vi "seguidor_parede_odometria.vi"(3 "Text":string, 4 "Line":i16(ring) items=["1", "2", "3", "4", "5", "6", "7", "8", "9", "10", "11", "12"], 5 "NXT/EV3 3":T1) -> (0 "Numeric 2":i32, 2 "NXT/EV3 2":T1)   [LabVIEW 2016]
uses:
  <vilib>/NXT/Subs/LVHSConnector.ctl
  <vilib>/NXT/LegoClasses/BrickReference/BrickReference.lvclass
  <vilib>/NXT/Block Support/NXT_OutputPort.ctl
  <vilib>/NXT/Block Support/NXT_InputPort.ctl
  <vilib>/NXT/Dual Mode Library/Motors/ResetMotor.vi
  <vilib>/NXT/NXTIO Xnodes/NXTIONodeSubVIs/NXTMoveMotors.vi
  <vilib>/NXT/Dual Mode Library/Sensors/EV3_Ultrasonic_CM.vi
  <vilib>/NXT/Dual Mode Library/Sensors/Touch_Pressed.vi
  <vilib>/NXT/Dual Mode Library/Motors/Rotation.vi
  <vilib>/NXT/Dual Mode Library/Display/drawText.vi
  <vilib>/NXT/Dual Mode Library/Display/drawNumber_float.vi
  <vilib>/NXT/NXTIO Xnodes/AddressXNode/NXTIOAddress.xnode
  <vilib>/NXT/NXTIO Xnodes/NXTIOXNode/NXTIO.xnode
panel:
  in  "KE 2":dbl=-0.0356
  in  "Kp":sgl
  in  "Dmin":sgl
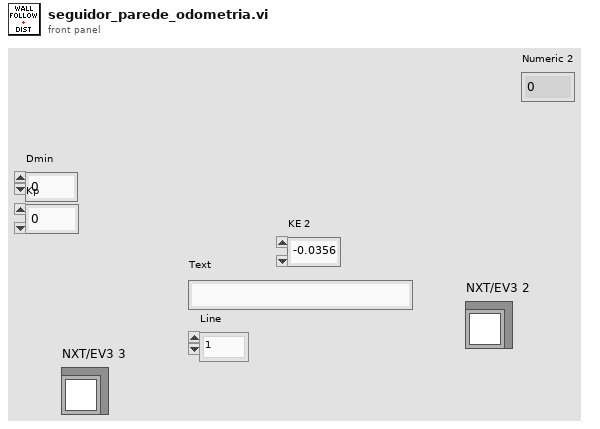
[diagram p1: front panel]
types:
  T1 = typedef "LVHSConnector.ctl" = refnum<class "BrickReference.lvclass">
  T2 = typedef "NXT_OutputPort.ctl" = u8
  T3 = typedef "NXT_InputPort.ctl" = u32
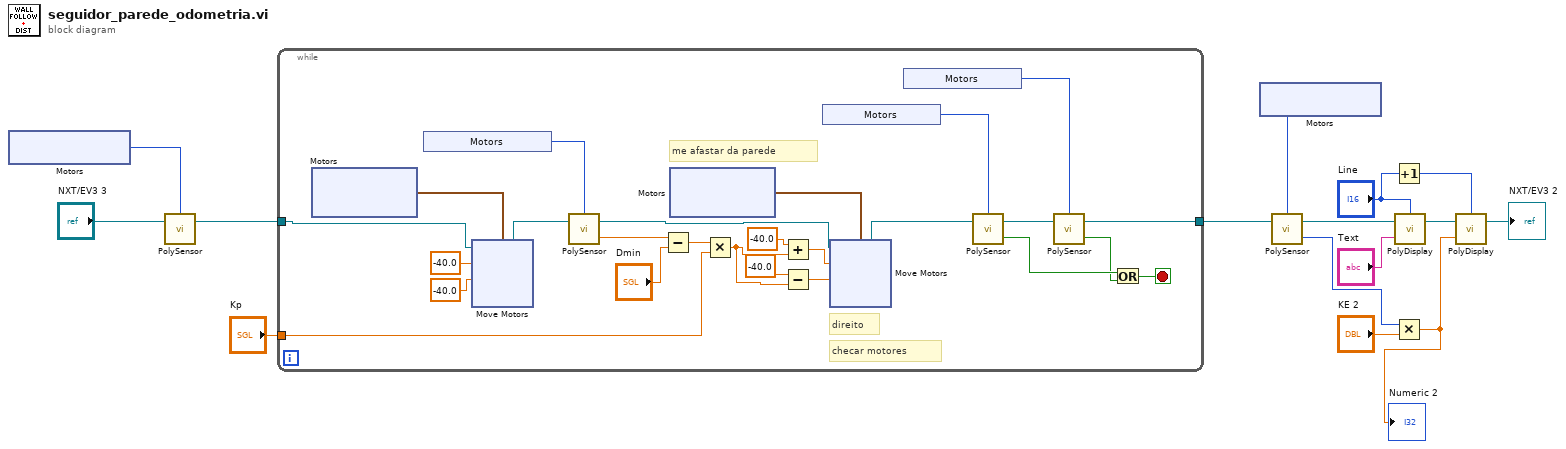
[diagram p0: block diagram]
diagram:
  n1 = xnode "Motors"() -> ("Motor"=w14:T2)
  n2 = call-poly <vilib>:"PolySensor.vi"("NXT/EV3"="NXT/EV3 3", "Port (All Ports)"=w14) -> ("NXT/EV3"=w12:T1)  [unwired: 2 out]
  n3 = while {
    tunnel: w12 -> [w37]
    tunnel: [w27] -> w2
    tunnel: "Kp" -> [w34]
    stop <- w24 stop-if-true
    # "direito"
    # "me afastar da parede"
    # "checar motores"
    n4 = xnode "Motors"() -> ("Motor"=w39:cluster{"Port":T2, "Port":T2})
    n5 = xnode "Motors"() -> ("Sensor"=w23:T3)
    n6 = xnode "Move Motors"("Power/Speed 2"=sgl -40.0 ("x"), "Power/Speed 1"=sgl -40.0 ("x"), "Motors"=w39, "NXT/EV3"=w37) -> ("NXT/EV3"=w38:T1)
    n7 = call-poly <vilib>:"PolySensor.vi"("NXT/EV3"=w38, "Port (Port 1)"=w23) -> ("Centimeters"=w19:sgl, "NXT/EV3"=w40:T1)  [unwired: 1 in]
    n8 = Subtract(x=w19, y="Dmin") -> (x-y=w32:sgl)
    n9 = xnode "Motors"() -> ("Motor"=w33:cluster{"Port":T2, "Port":T2})
    n10 = Multiply(x=w32, y=w34) -> (x*y=w16:sgl)
    n11 = Add(x=sgl -40.0, y=w16) -> (x+y=w30:sgl)
    n12 = Subtract(x=sgl -40.0, y=w16) -> (x-y=w31:sgl)
    n13 = xnode "Motors"() -> ("Sensor"=w22:T3)
    n14 = xnode "Move Motors"("Power/Speed 2"=w31, "Power/Speed 1"=w30, "Motors"=w33, "NXT/EV3"=w40) -> ("NXT/EV3"=w28:T1)
    n15 = xnode "Motors"() -> ("Sensor"=w21:T3)
    n16 = call-poly <vilib>:"PolySensor.vi"("NXT/EV3"=w28, "Port (Port 1)"=w22) -> ("Yes / No"=w26:bool, "NXT/EV3"=w29:T1)  [unwired: 1 in]
    n17 = call-poly <vilib>:"PolySensor.vi"("NXT/EV3"=w29, "Port (Port 1)"=w21) -> ("Yes / No"=w25:bool, "NXT/EV3"=w27:T1)  [unwired: 1 in]
    n18 = Or(x=w26, y=w25) -> (x .or. y?=w24:bool)
  }
  n19 = xnode "Motors"() -> ("Motor"=w11:T2)
  n20 = call-poly <vilib>:"PolySensor.vi"("NXT/EV3"=w2, "Port (Port A)"=w11) -> ("Angle of Rotation"=w8:i32, "NXT/EV3"=w7:T1)  [unwired: 1 out]
  n21 = Increment(x="Line") -> (x+1=w3:i16)
  n22 = Multiply(x=w8, y="KE 2") -> (x*y=w1:dbl)
  "Numeric 2" <- w1
  n23 = call-poly <vilib>:"PolyDisplay.vi"("Text"="Text", "NXT/EV3"=w7, "Line"="Line") -> ("NXT/EV3"=w6:T1)  [unwired: 1 in]
  n24 = call-poly <vilib>:"PolyDisplay.vi"("number"=w1, "NXT/EV3"=w6, "Line"=w3) -> ("NXT/EV3"=→"NXT/EV3 2":T1)  [unwired: 1 in]
